vi "From String.vi"(0 "Value":string, 1 "Key":string) -> (2 "Map":refnum<class "Map.lvclass">)   [LabVIEW 2018, in "Toolkit.lvlib" / "Data.lvlib" / "Map.lvclass"]
uses:
  Map.lvclass
  Map.lvclass/Map.ctl
  String/String.lvclass
  D:/Users/cfield/Code/Field R&D Services/Mustache/LabVIEW/trunk/src/Toolkit/Data/Abstract/Abstract.lvclass
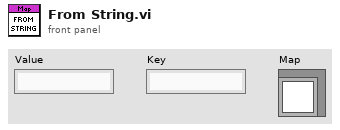
[diagram p1: front panel]
types:
  T1 = cluster{"Key":string, "String":refnum<class "String.lvclass">}
  T2 = cluster{"Key":string, "String":refnum<class "String.lvclass">}[]
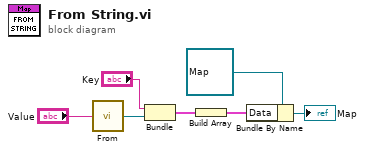
[diagram p0: block diagram]
diagram:
  n1 = call "From.vi"("Value"="Value") -> ("String"=w1:refnum<class "String.lvclass">)
  n2 = Bundle("Key"="Key", "String"=w1) -> (w4:T1)  [unwired: 1 in]
  n3 = Build Array(w4) -> (w3:T2)
  n4 = Bundle By Name(cluster=refnum<class "Map.lvclass"> refnum ("Toolkit.lvlib:Data.lvlib:Map.lvclass"), "Data"=w3) -> (→"Map":refnum<class "Map.lvclass">)
